vi "Get Enqueuer.vi"(7 "Enqueuer Ident":string, 8 "error in (no error)":errorcluster, 11 "My Actor in":refnum<class "My Actor.lvclass">) -> (0 "error out":errorcluster, 2 "Nested Actor's Enqueuer":refnum<class "Message Enqueuer.lvclass">, 3 "My Actor out":refnum<class "My Actor.lvclass">)   [LabVIEW 2023, in "My Actor.lvlib" / "My Actor.lvclass"]
uses:
  My Actor.lvclass
  <vilib>/ActorFramework/Message Enqueuer/Message Enqueuer.lvclass
  My Actor.lvclass/My Actor.ctl
  <vilib>/Utility/error.llb/Error Cluster From Error Code.vi
  <vilib>/ErrorRing/Error Ring.xnode
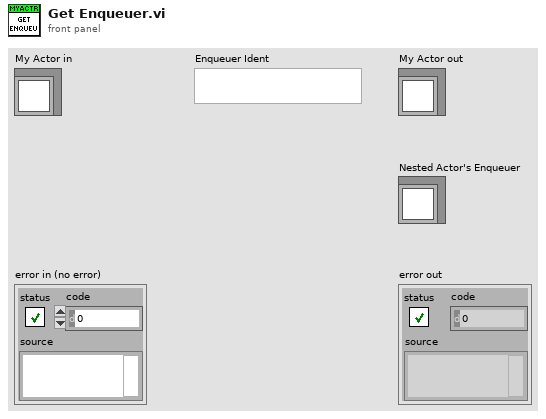
[diagram p1: front panel]
types:
  T1 = map{string, refnum<class "Message Enqueuer.lvclass">}
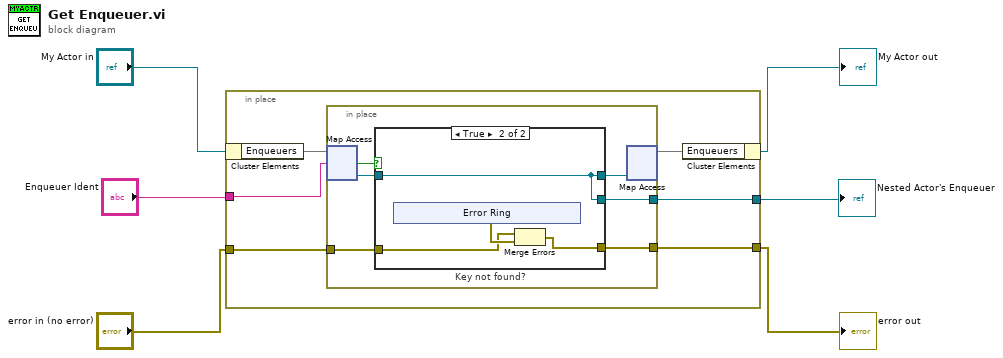
[diagram p0: block diagram]
diagram:
  n1 = in-place {
    in-place-border: "Enqueuer Ident" -> [w11]
    in-place-border: "error in (no error)" -> [w10]
    in-place-border: [w9] -> w1
    in-place-border: [w8] -> w4
    n2 = in-place-cluster #1("My Actor in") -> ("Enqueuers"=w12:T1)
    n3 = in-place {
      in-place-border: w10 -> [w18]
      in-place-border: [w17] -> w9
      in-place-border: [w14] -> w8
      n4 = in-place-map #2(w12, w11) -> (w16:refnum<class "Message Enqueuer.lvclass">, w13:bool)  [unwired: 1 in]
      n5 = case "Key not found?" shown="True" w13 {
        tunnel: w18 -> [w19 w23]
        tunnel: [w19 w22] -> w17
        tunnel: w16 -> [w20 w21]
        tunnel: [w20 w21] -> w15
        tunnel: [w20 w21] -> w14
        frame False {
        }
        frame True {
          n6 = xnode "Error Ring"() -> ("error out"=w24:errorcluster)
          n7 = Merge Errors(w23, w24) -> (w22:errorcluster)
        }
      }
      n8 = in-place-map #2(w15) -> (w7:T1)  [unwired: 1 in, 2 out]
    }
    n9 = in-place-cluster #1("Enqueuers"=w7) -> (→"My Actor out":refnum<class "My Actor.lvclass">)
  }
  "error out" <- w1
  "Nested Actor's Enqueuer" <- w4
